vi "OverlayLines.vi"(11 "Image":T1) -> (3 "Image Out":T1)   [LabVIEW 2015]
uses:
  <vilib>/vision/Image Controls.llb/IMAQ Image.ctl
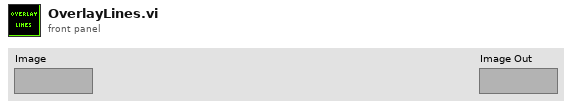
[diagram p1: front panel]
types:
  T1 = typedef "IMAQ Image.ctl" = refnum<image>
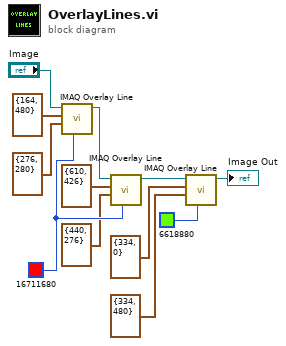
[diagram p0: block diagram]
diagram:
  w8 = u32 16711680 ("Color")
  n1 = call "IMAQ Overlay Line"("Color"=w8, "End Point"=cluster{"X":i32, "Y":i32} {"X"=276, "Y"=280}, "Start Point"=cluster{"X":i32, "Y":i32} {"X"=164, "Y"=480}, "Image"="Image") -> ("Image Out"=w9:T1)  [unwired: 6 in, 1 out]
  n2 = call "IMAQ Overlay Line"("Color"=w8, "End Point"=cluster{"X":i32, "Y":i32} {"X"=440, "Y"=276}, "Start Point"=cluster{"X":i32, "Y":i32} {"X"=610, "Y"=426}, "Image"=w9) -> ("Image Out"=w5:T1)  [unwired: 6 in, 1 out]
  n3 = call "IMAQ Overlay Line"("Color"=u32 6618880, "End Point"=cluster{"X":i32, "Y":i32} {"X"=334, "Y"=480}, "Start Point"=cluster{"X":i32, "Y":i32} {"X"=334, "Y"=0}, "Image"=w5) -> ("Image Out"=→"Image Out":T1)  [unwired: 6 in, 1 out]
